vi "GTCP331-200ER - 1.C.(2).vi"(8 "error in (no error)":errorcluster, 11 "RT - Analysis Data in in in":T1={"Accel Sensistivity"=[0.0, 0.0, 0.0], "Cutoff Frequncies"=[{"LP Passband"=0.0, "HP Stopband"=0.0, "LP Stopband"=0.0, "HP Passband"=0.0}, {"LP Passband"=0.0, "HP Stopband"=0.0, "LP Stopband"=0.0, "HP Passband"=0.0}, {"LP Passband"=0.0, "HP Stopband"=0.0, "LP Stopband"=0.0, "HP Passband"=0.0}], "APU Setup File"={"Sensor Info"=[], "Calibration Info"=[], "CMM Table 106"=[], "CMM Table 106B "=[], "Accel Config"=[], "Report Sheet 1"=[], "Report Sheet 2"=[], "Report Sheet 3"=[]}, "RepairLevel"=""} {"Cutoff Frequncies"."HP Passband" min=1.0 step=1.0 format="%#.4f"; "Cutoff Frequncies"."LP Stopband" min=1.0 step=1.0 format="%#.4f"; "Cutoff Frequncies"."HP Stopband" min=1.0 step=1.0 format="%#.4f"; "Cutoff Frequncies"."LP Passband" min=1.0 step=1.0 format="%#.4f"}) -> (0 "error out":errorcluster, 2 "Interactive Mode Vals":dbl[](array[numeric]), 3 "RT - Analysis Data in out":T1 {"Cutoff Frequncies"."HP Passband" min=1.0 step=1.0 format="%#.4f"; "Cutoff Frequncies"."LP Stopband" min=1.0 step=1.0 format="%#.4f"; "Cutoff Frequncies"."HP Stopband" min=1.0 step=1.0 format="%#.4f"; "Cutoff Frequncies"."LP Passband" min=1.0 step=1.0 format="%#.4f"})   [LabVIEW 2018, in "RT - Analysis.lvlib"]
doc: "This subtest perfmors engine run-in procedures."
uses:
  RT - Analysis.lvlib
  Private Controls/Watchdog Settings.ctl
  Public Controls/Alert Data.ctl
  Private Controls/RT-Analysis Data.ctl
  Modules/Testing UI 3/Private Controls/Cutoff Frequency.ctl
  Modules/Testing UI 3/Testing UI 3.lvlib
  Top Level/Shared Controls/APU Setup File.ctl
panel:
  # "Highpass Cutoff Frequency"
  # "Lowpass Cutoff Frequency"
  # "Highpass Cutoff Frequency"
  # "Lowpass Cutoff Frequency"
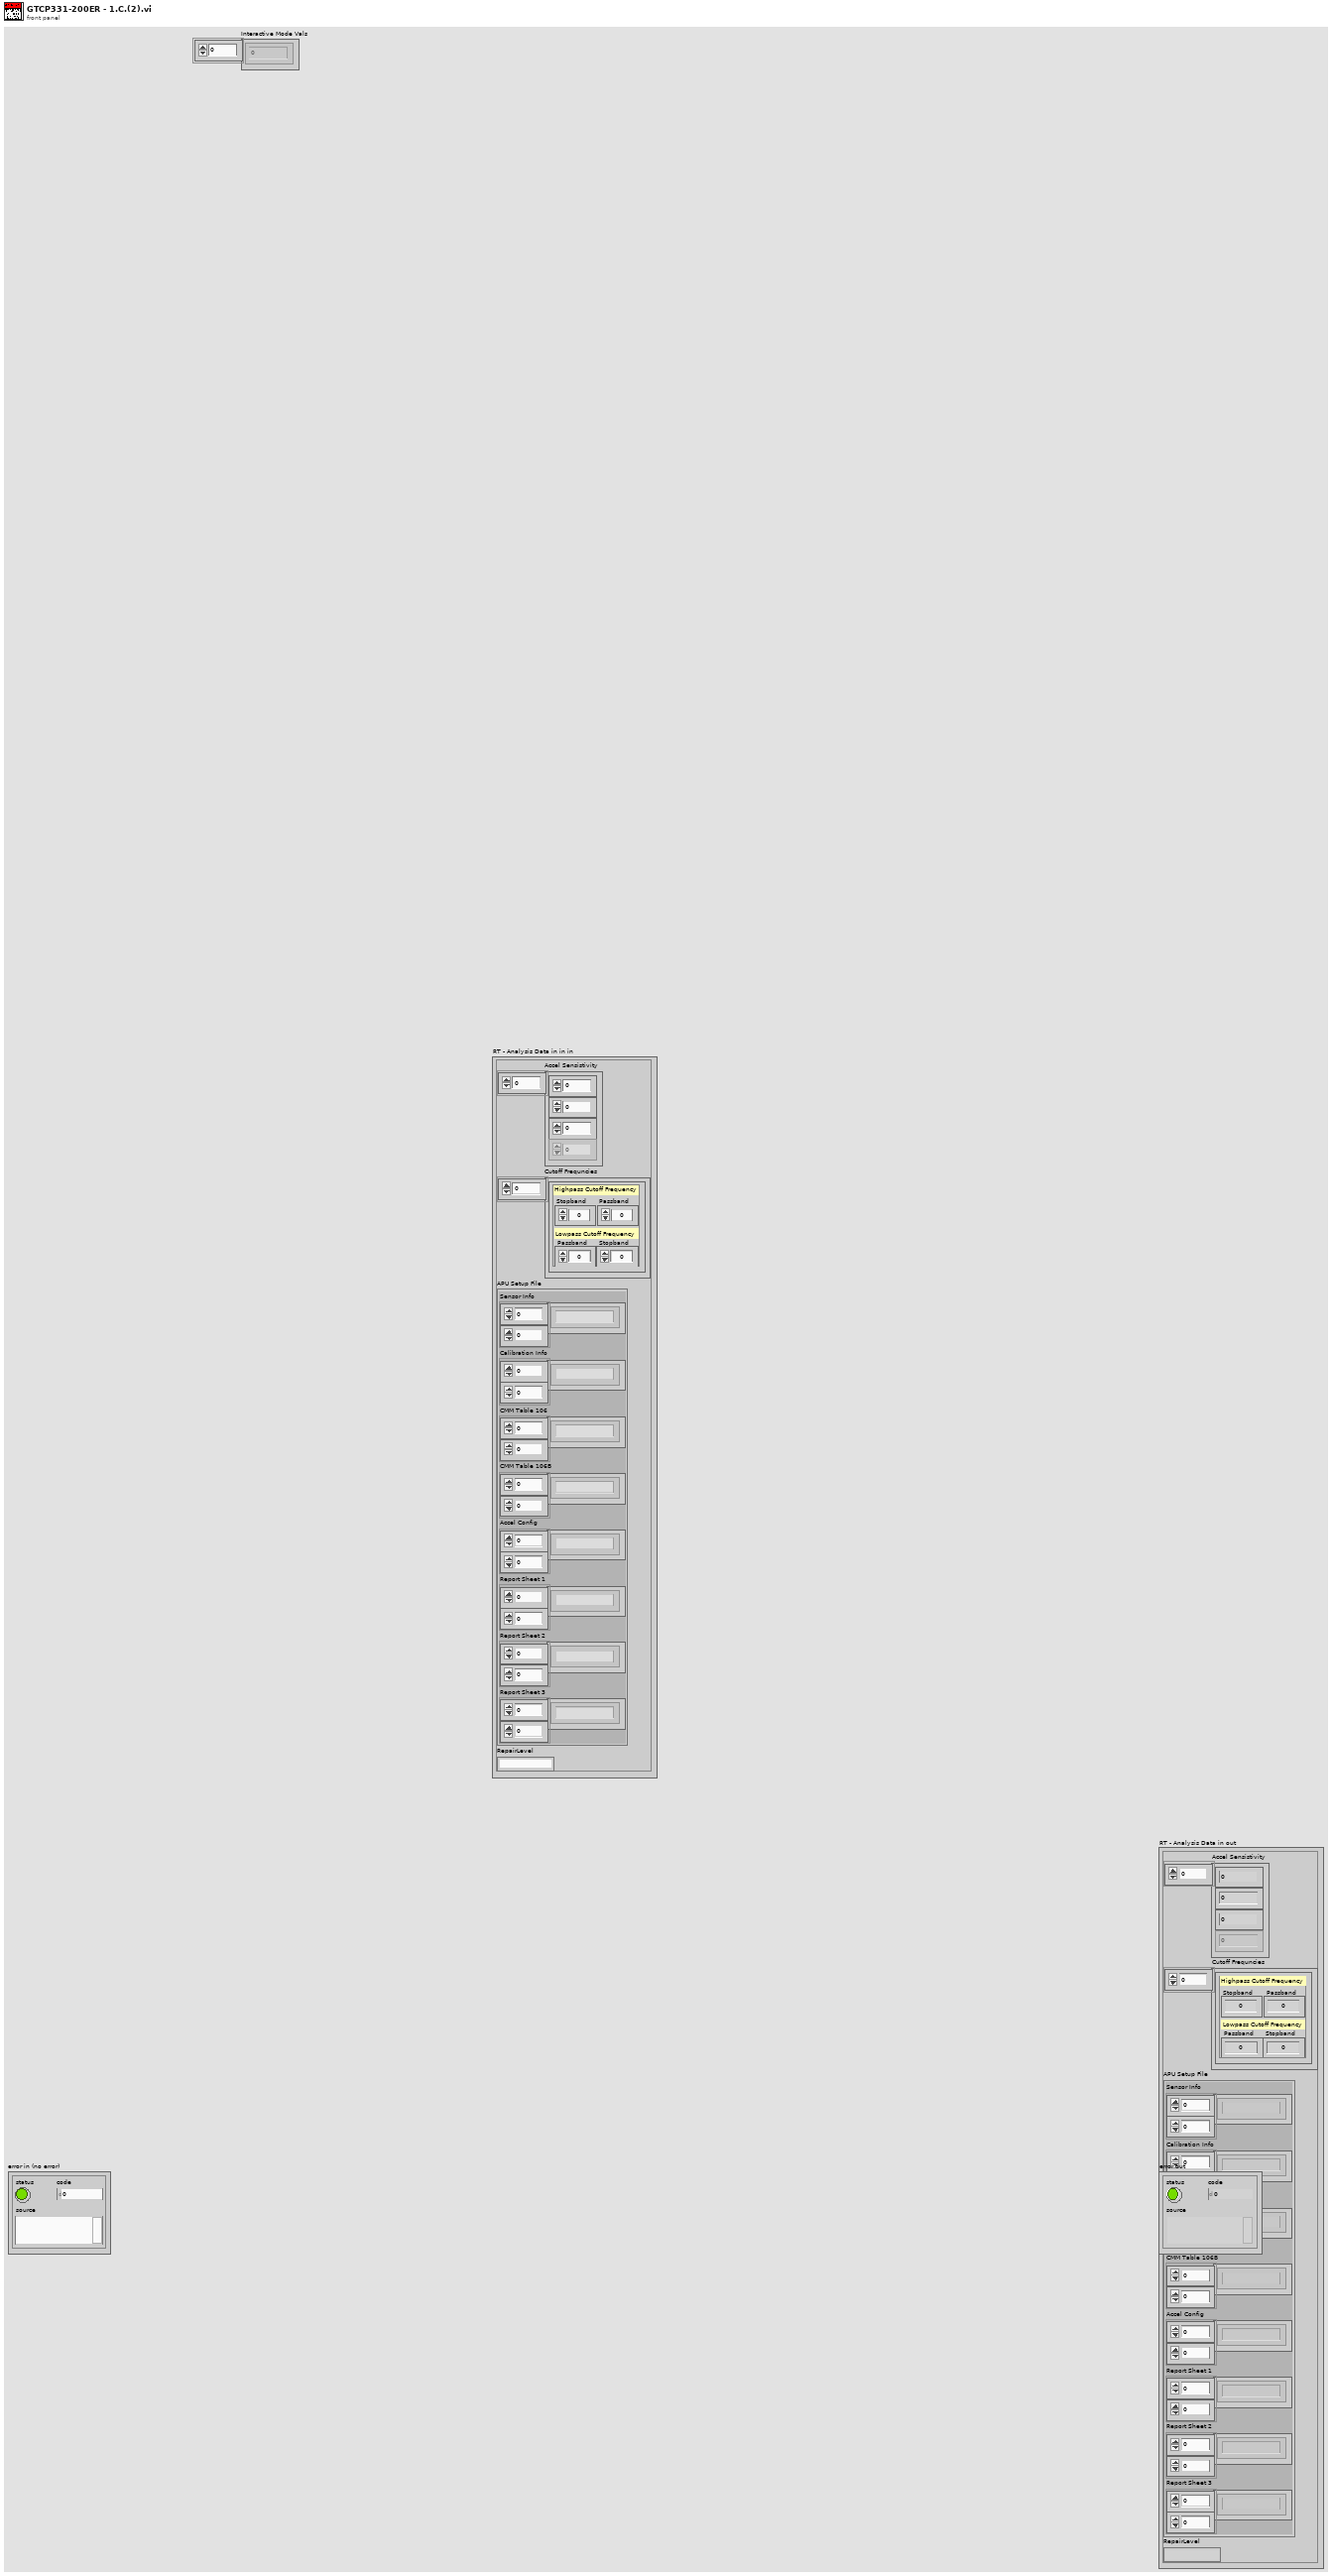
[diagram p1: front panel]
types:
  T1 = typedef "RT - Analysis.lvlib/RT-Analysis Data.ctl" = cluster{"Accel Sensistivity":dbl[], "Cutoff Frequncies":T2[], "APU Setup File":T3, "RepairLevel":string}
  T2 = typedef "Testing UI 3.lvlib/Cutoff Frequency.ctl" = cluster{"LP Passband":dbl, "HP Stopband":dbl, "LP Stopband":dbl, "HP Passband":dbl}
  T3 = typedef "APU Setup File.ctl" = cluster{"Sensor Info":string[][], "Calibration Info":string[][], "CMM Table 106":string[][], "CMM Table 106B ":string[][], "Accel Config":string[][], "Report Sheet 1":string[][], "Report Sheet 2":string[][], "Report Sheet 3":string[][]}
  T4 = typedef "RT - Analysis.lvlib/Alert Data.ctl" = cluster{"Tag":string, "Value":dbl, "Alerts":bool[], "Thresh Val":dbl, "Thresh Len":dbl, "Thresh Type":enum16{"Neither", "Max", "Min"}}
  T5 = typedef "RT - Analysis.lvlib/Watchdog Settings.ctl" = cluster{"Watchdog Action":enum16{"Disabled", "Timer - Change Sample Rate", "RPM Thresh - Insert Other", "RPM Thresh - Check POPD", "RPM Thresh - StartStop Logging"}, "Timer Start":timestamp, "[Watchdog Bools]":bool[], "[Watchdog DBLs]":dbl[], "Watchdog Variant":variant}
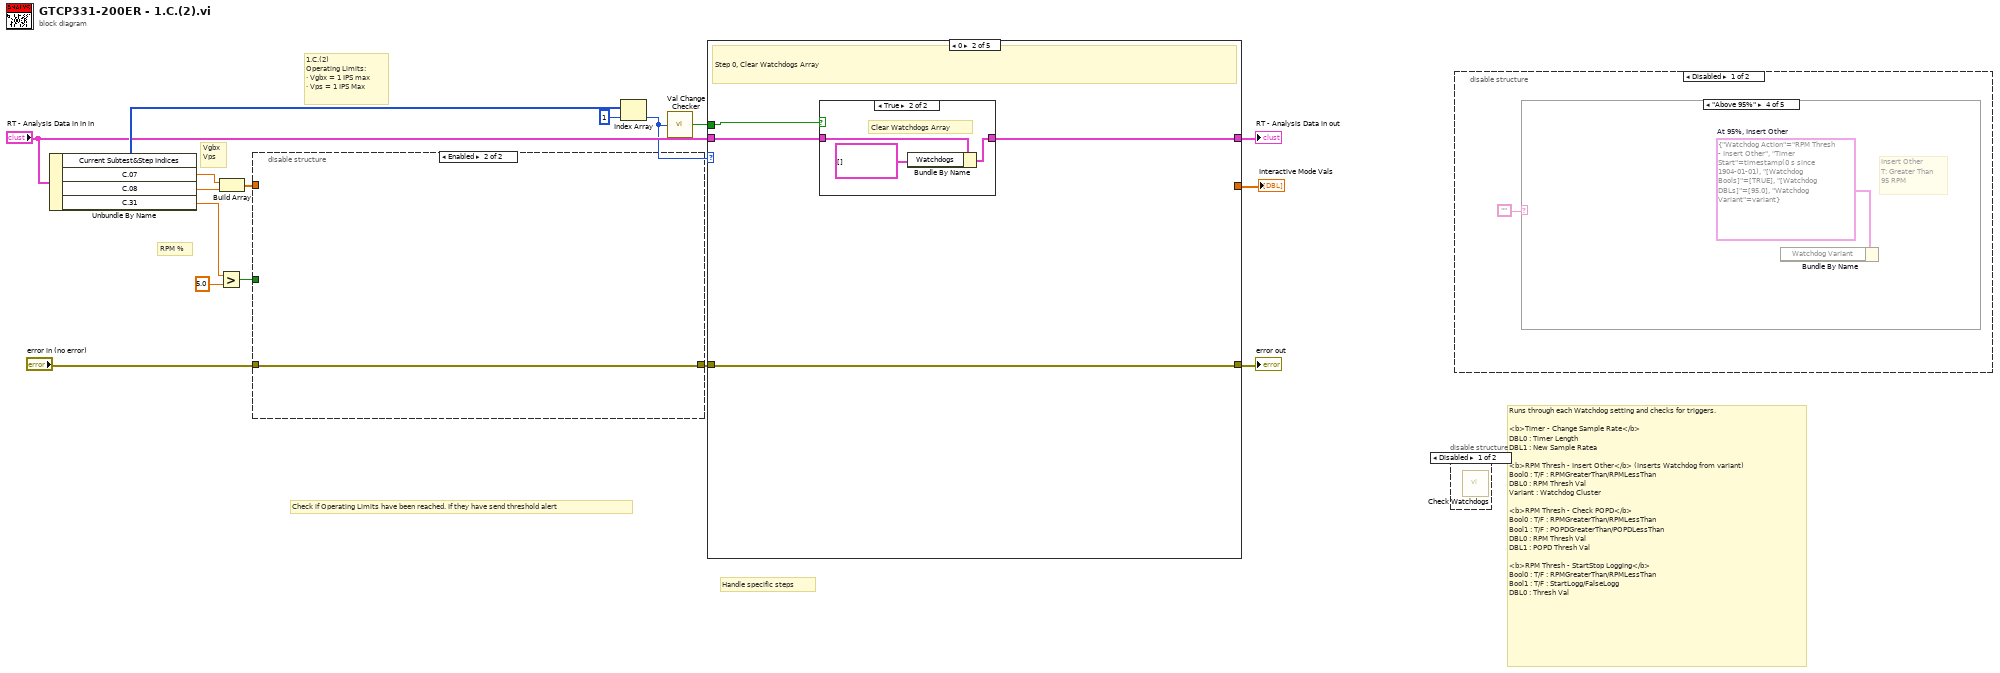
[diagram p0: block diagram]
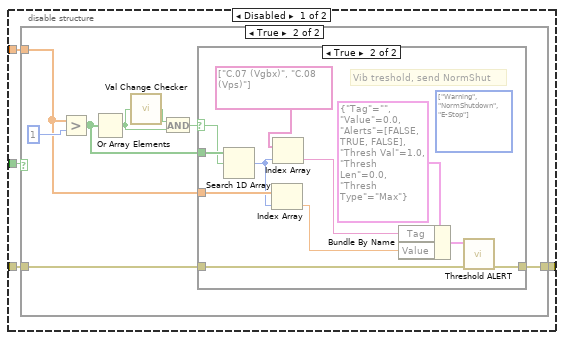
[diagram p2: hidden frame]
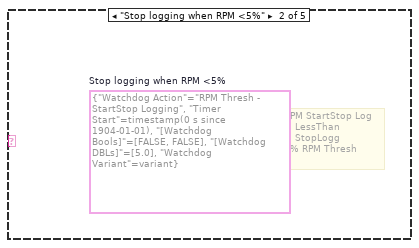
[diagram p6: hidden frame]
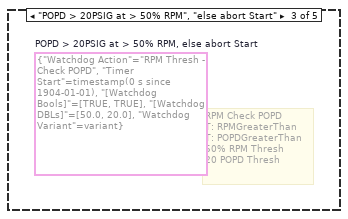
[diagram p7: hidden frame]
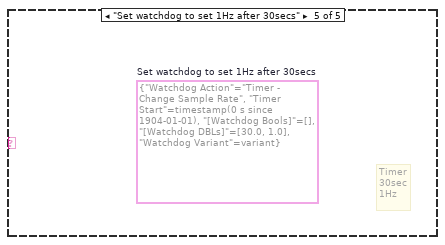
[diagram p8: hidden frame]
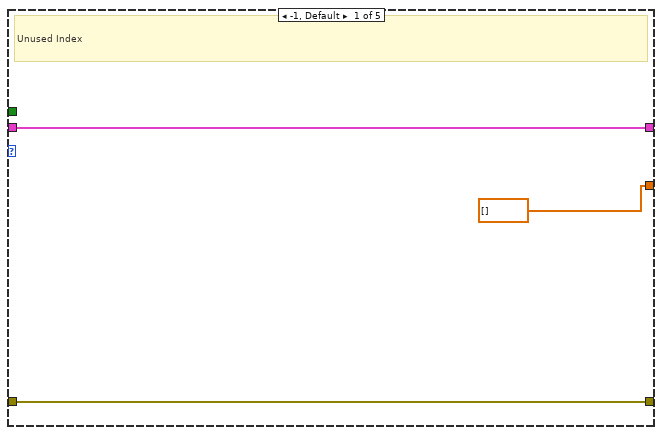
[diagram p11: hidden frame]
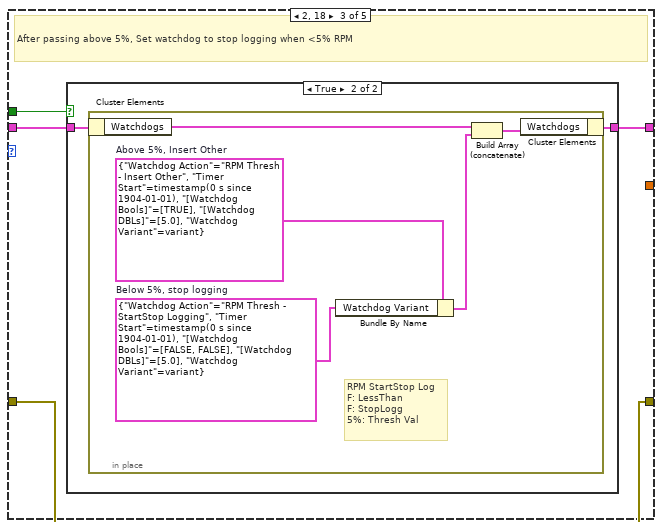
[diagram p13: hidden frame]
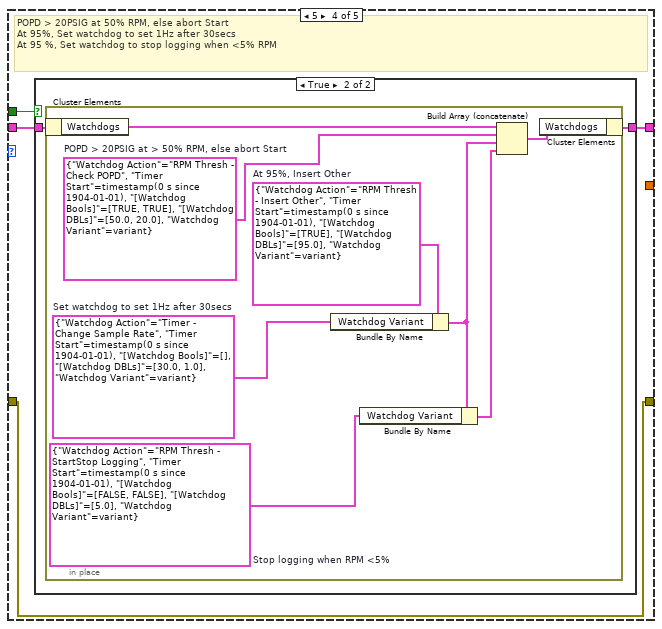
[diagram p15: hidden frame]
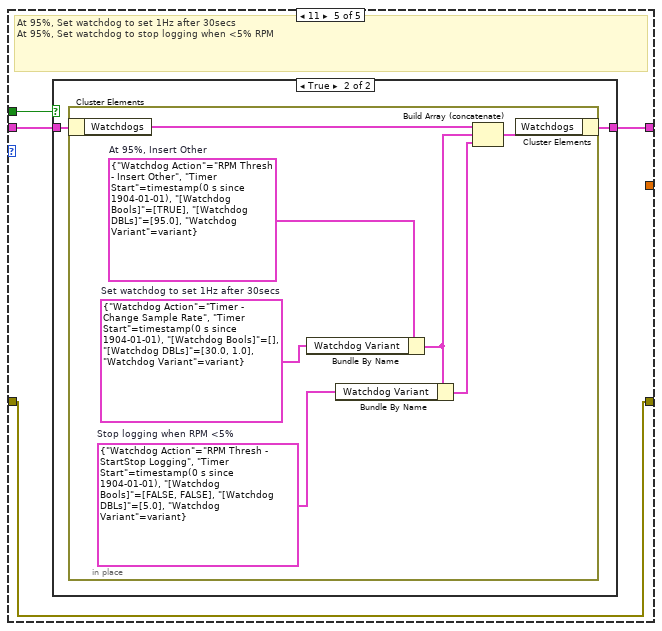
[diagram p17: hidden frame]
diagram:
  # "Handle specific steps"
  # "RPM %"
  # "Runs through each Watchdog setting and checks for triggers.\n\n<b>Timer - Change Sample Rate</b>\nDBL0 : Timer Length\nDBL1 : New Sample Ratea\n\n<b>RPM Thresh - Insert Other</b> (Inserts Watchdog from variant)\nBool0 : T/F : RPMGreaterThan/RPMLessThan\nDBL0 : RPM Thresh Val\nVariant : Watchdog Cluster\n\n<b>RPM Thresh - Check POPD</b>\nBool0 : T/F : RPMGreaterThan/RPMLessThan\nBool1 : T/F : POPDGreaterThan/POPDLessThan\nDBL0 : RPM Thresh Val\nDBL1 : POPD Thresh Val\n\n<b>RPM Thresh - StartStop Logging</b>\nBool0 : T/F : RPMGreaterThan/RPMLessThan\nBool1 : T/F : StartLogg/FalseLogg\nDBL0 : Thresh Val"
  # "Check if Operating Limits have been reached. If they have send threshold alert"
  # "Vgbx\nVps"
  # "1.C.(2)\nOperating Limits:\n· Vgbx = 1 IPS max\n· Vps = 1 IPS Max"
  n1 = Unbundle By Name("RT - Analysis Data in in in") -> ("Current Subtest&Step Indices"=w16:i32[], "C.07"=w11:dbl, "C.08"=w10:dbl, "C.31"=w2:dbl)
  n2 = Greater?(x=w2, y=5.0) -> (0:w3:bool)
  n3 = Build Array(w11, w10) -> (w1:dbl[])
  n4 = disable-structure shown="Enabled" {
    disable-tunnel: [w20 w42] -> w5
    disable-tunnel: "error in (no error)" -> [w19 w42]
    disable-tunnel: w3 -> [w18 _]
    disable-tunnel: w1 -> [w17 _]
    frame Disabled {
      n5 = case shown="True" w18 {
        tunnel: [w21 w28] -> w20
        tunnel: w17 -> [_ w26]
        tunnel: w19 -> [w21 w22]
        frame False {
        }
        frame True {
          n6 = Greater?(x=w26, y=1 ("C.08")) -> (0:w27:bool[])
          n7 = Or Array Elements(Boolean array=w27) -> (logical OR=w24:bool)
          n8 = call "Val Change Checker.vi"("Current Value in"=w24) -> ("Value Change?"=w25:bool)
          n9 = And(x=w25, y=w24) -> (x .and. y?=w23:bool)
          n10 = case shown="True" w23 {
            selector: w23 -> [_ w40]
            tunnel: w22 -> [w30 w36]
            tunnel: [w30 w35] -> w28
            tunnel: w27 -> [_ w41]
            tunnel: w26 -> [_ w39]
            frame False {
            }
            frame True {
              (unwired) enum32{"Warning", "NormShutdown", "E-Stop"}[] [enum."Warning", enum."NormShutdown", enum."E-Stop"] items=["Warning", "NormShutdown", "E-Stop"]
              # "Vib treshold, send NormShut"
              n11 = Search 1D Array(1D array=w41, element=w40) -> (index of element=w38:i32)  [unwired: 1 in]
              n12 = Index Array(array=w39, index=w38) -> (element=w31:dbl)
              n13 = Index Array(array=string[] ["C.07 (Vgbx)", "C.08 (Vps)"], index=w38) -> (element=w32:string)
              n14 = Bundle By Name(cluster=T4 {"Tag"="", "Value"=0.0, "Alerts"=[FALSE, TRUE, FALSE], "Thresh Val"=1.0, "Thresh Len"=0.0, "Thresh Type"=enum."Max"} ("Alert Data"), "Tag"=w32, "Value"=w31) -> (w34:T4)
              n15 = call "Threshold ALERT.vi"("error in (no error)"=w36, "Alert Data"=w34) -> ("error out"=w35:errorcluster)  [unwired: 9 in]
            }
          }
        }
      }
    }
    frame Enabled {
    }
  }
  n16 = Index Array(array=w16, index=1) -> (element=w8:i32)
  n17 = call "Val Change Checker.vi"("Current Value in"=w8) -> ("Value Change?"=w7:bool)
  n18 = case shown="0" w8 {
    tunnel: [w45 w46 w57 w69 w84] -> w14
    tunnel: w5 -> [w45 w46 w57 w69 w84]
    tunnel: [w44 w48 w56 w68 w83] -> w13
    tunnel: "RT - Analysis Data in in in" -> [w44 w49 w55 w67 w82]
    tunnel: [dbl[] [] ("Interactive Mode Vals") _ _ _ _] -> w12
    tunnel: w7 -> [_ w47 w54 w66 w81]
    frame -1, Default {
      # "Unused Index"
    }
    frame 0 {
      # "Step 0, Clear Watchdogs Array"
      n19 = case shown="True" w47 {
        tunnel: w49 -> [w50 w53]
        tunnel: [w50 w52] -> w48
        frame False {
        }
        frame True {
          # "Clear Watchdogs Array"
          n20 = Bundle By Name(cluster=w53, "Watchdogs"=T5[] []) -> (w52:T1)
        }
      }
    }
    frame 2, 18 {
      # "After passing above 5%, Set watchdog to stop logging when <5% RPM"
      n21 = case shown="True" w54 {
        tunnel: [w58 w60] -> w56
        tunnel: w55 -> [w58 w59]
        frame False {
        }
        frame True {
          n22 = in-place {
            w61 = T5 {"Watchdog Action"=enum."RPM Thresh - StartStop Logging", "Timer Start"=timestamp(0 s since 1904-01-01), "[Watchdog Bools]"=[FALSE, FALSE], "[Watchdog DBLs]"=[5.0], "Watchdog Variant"=variant}  # Below 5%, stop logging
            w63 = T5 {"Watchdog Action"=enum."RPM Thresh - Insert Other", "Timer Start"=timestamp(0 s since 1904-01-01), "[Watchdog Bools]"=[TRUE], "[Watchdog DBLs]"=[5.0], "Watchdog Variant"=variant}  # Above 5%, Insert Other
            # "RPM StartStop Log\nF: LessThan\nF: StopLogg\n5%: Thresh Val"
            n23 = in-place-cluster #1(w59) -> ("Watchdogs"=w64:T5[])
            n24 = Bundle By Name(cluster=w63, "Watchdog Variant"=w61) -> (w62:T5)
            n25 = Build Array (concatenate)(w64, w62) -> (w65:T5[])
            n26 = in-place-cluster #1("Watchdogs"=w65) -> (w60:T1)
          }
        }
      }
    }
    frame 5 {
      # "POPD > 20PSIG at 50% RPM, else abort Start\nAt 95%, Set watchdog to set 1Hz after 30secs\nAt 95 %, Set watchdog to stop logging when <5% RPM"
      n27 = case shown="True" w66 {
        tunnel: [w70 w72] -> w68
        tunnel: w67 -> [w70 w71]
        frame False {
        }
        frame True {
          n28 = in-place {
            w73 = T5 {"Watchdog Action"=enum."RPM Thresh - StartStop Logging", "Timer Start"=timestamp(0 s since 1904-01-01), "[Watchdog Bools]"=[FALSE, FALSE], "[Watchdog DBLs]"=[5.0], "Watchdog Variant"=variant}  # Stop logging when RPM <5%
            w78 = T5 {"Watchdog Action"=enum."Timer - Change Sample Rate", "Timer Start"=timestamp(0 s since 1904-01-01), "[Watchdog Bools]"=[], "[Watchdog DBLs]"=[30.0, 1.0], "Watchdog Variant"=variant}  # Set watchdog to set 1Hz after 30secs
            w77 = T5 {"Watchdog Action"=enum."RPM Thresh - Insert Other", "Timer Start"=timestamp(0 s since 1904-01-01), "[Watchdog Bools]"=[TRUE], "[Watchdog DBLs]"=[95.0], "Watchdog Variant"=variant}  # At 95%, Insert Other
            w76 = T5 {"Watchdog Action"=enum."RPM Thresh - Check POPD", "Timer Start"=timestamp(0 s since 1904-01-01), "[Watchdog Bools]"=[TRUE, TRUE], "[Watchdog DBLs]"=[50.0, 20.0], "Watchdog Variant"=variant}  # POPD > 20PSIG at > 50% RPM, else abort Start
            n29 = in-place-cluster #2(w71) -> ("Watchdogs"=w79:T5[])
            n30 = Bundle By Name(cluster=w77, "Watchdog Variant"=w78) -> (w75:T5)
            n31 = Bundle By Name(cluster=w75, "Watchdog Variant"=w73) -> (w74:T5)
            n32 = Build Array (concatenate)(w79, w76, w75, w74) -> (w80:T5[])
            n33 = in-place-cluster #2("Watchdogs"=w80) -> (w72:T1)
          }
        }
      }
    }
    frame 11 {
      # "At 95%, Set watchdog to set 1Hz after 30secs\nAt 95%, Set watchdog to stop logging when <5% RPM"
      n34 = case shown="True" w81 {
        tunnel: [w85 w87] -> w83
        tunnel: w82 -> [w85 w86]
        frame False {
        }
        frame True {
          n35 = in-place {
            w88 = T5 {"Watchdog Action"=enum."RPM Thresh - StartStop Logging", "Timer Start"=timestamp(0 s since 1904-01-01), "[Watchdog Bools]"=[FALSE, FALSE], "[Watchdog DBLs]"=[5.0], "Watchdog Variant"=variant}  # Stop logging when RPM <5%
            w92 = T5 {"Watchdog Action"=enum."Timer - Change Sample Rate", "Timer Start"=timestamp(0 s since 1904-01-01), "[Watchdog Bools]"=[], "[Watchdog DBLs]"=[30.0, 1.0], "Watchdog Variant"=variant}  # Set watchdog to set 1Hz after 30secs
            w91 = T5 {"Watchdog Action"=enum."RPM Thresh - Insert Other", "Timer Start"=timestamp(0 s since 1904-01-01), "[Watchdog Bools]"=[TRUE], "[Watchdog DBLs]"=[95.0], "Watchdog Variant"=variant}  # At 95%, Insert Other
            n36 = in-place-cluster #3(w86) -> ("Watchdogs"=w93:T5[])
            n37 = Bundle By Name(cluster=w91, "Watchdog Variant"=w92) -> (w90:T5)
            n38 = Bundle By Name(cluster=w90, "Watchdog Variant"=w88) -> (w89:T5)
            n39 = Build Array (concatenate)(w93, w90, w89) -> (w94:T5[])
            n40 = in-place-cluster #3("Watchdogs"=w94) -> (w87:T1)
          }
        }
      }
    }
  }
  "RT - Analysis Data in out" <- w13
  "error out" <- w14
  "Interactive Mode Vals" <- w12
  n41 = disable-structure shown="Disabled" {
    frame Disabled {
      n42 = call "Check Watchdogs.vi"() -> ()  [unwired: 10 in, 2 out]
    }
    frame Enabled {
    }
  }
  n43 = disable-structure shown="Disabled" {
    frame Disabled {
      n44 = case shown="\"Above 95%\"" "" {
        frame Default {
        }
        frame "Stop logging when RPM <5%" {
          (unwired) T5 {"Watchdog Action"=enum."RPM Thresh - StartStop Logging", "Timer Start"=timestamp(0 s since 1904-01-01), "[Watchdog Bools]"=[FALSE, FALSE], "[Watchdog DBLs]"=[5.0], "Watchdog Variant"=variant}  # Stop logging when RPM <5%
          # "RPM StartStop Log\nF: LessThan\nF: StopLogg\n5% RPM Thresh"
        }
        frame "POPD > 20PSIG at > 50% RPM", "else abort Start" {
          (unwired) T5 {"Watchdog Action"=enum."RPM Thresh - Check POPD", "Timer Start"=timestamp(0 s since 1904-01-01), "[Watchdog Bools]"=[TRUE, TRUE], "[Watchdog DBLs]"=[50.0, 20.0], "Watchdog Variant"=variant}  # POPD > 20PSIG at > 50% RPM, else abort Start
          # "RPM Check POPD\nT: RPMGreaterThan\nT: POPDGreaterThan\n50% RPM Thresh\n20 POPD Thresh"
        }
        frame "Above 95%" {
          w96 = T5 {"Watchdog Action"=enum."RPM Thresh - Insert Other", "Timer Start"=timestamp(0 s since 1904-01-01), "[Watchdog Bools]"=[TRUE], "[Watchdog DBLs]"=[95.0], "Watchdog Variant"=variant}  # At 95%, Insert Other
          # "Insert Other\nT: Greater Than\n95 RPM"
          n45 = Bundle By Name(cluster=w96) -> ()  [unwired: 1 in, 1 out]
        }
        frame "Set watchdog to set 1Hz after 30secs" {
          (unwired) T5 {"Watchdog Action"=enum."Timer - Change Sample Rate", "Timer Start"=timestamp(0 s since 1904-01-01), "[Watchdog Bools]"=[], "[Watchdog DBLs]"=[30.0, 1.0], "Watchdog Variant"=variant}  # Set watchdog to set 1Hz after 30secs
          # "Timer\n30sec\n1Hz"
        }
      }
    }
    frame Enabled {
    }
  }
